vi "GetWirelessEndpointAuths.vi"(8 "error in (no error)":errorcluster) -> (0 "error out":errorcluster, 1 "found":bool, 3 "wireless endpoint auths":T1[](array[typedef]))   [LabVIEW 2017, in "GlobalConfiguration.lvlib"]
uses:
  <vilib>/addons/InsightCM/Utilities/GlobalConfiguration/GlobalConfiguration.lvlib
  <vilib>/addons/InsightCM/MessageBus/Base/controls/WirelessEndpointAuth.ctl
  <vilib>/addons/PointValueMap/subVIs/Point_Read_variant.vi
  <vilib>/addons/PointValueMap/subVIs/Point_Write_variant.vi
  <vilib>/addons/PointValueMap/PointValueMap.lvlib
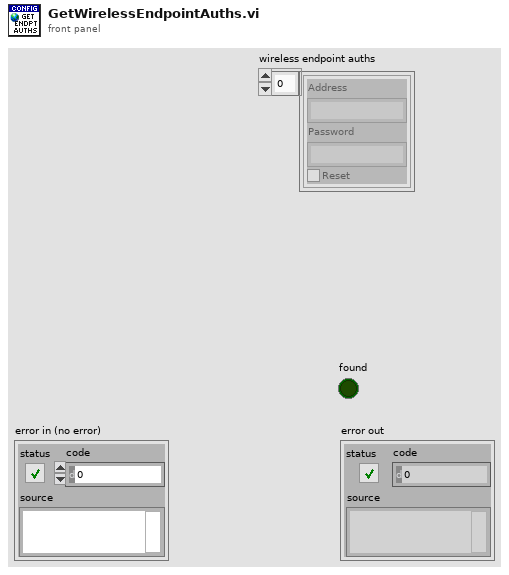
[diagram p1: front panel]
types:
  T1 = typedef "WirelessEndpointAuth.ctl" = cluster{"Address":string, "Password":string, "Reset":bool}
  T2 = typedef "PointValueMap.lvlib/PointMap.ctl" = refnum<data-value>
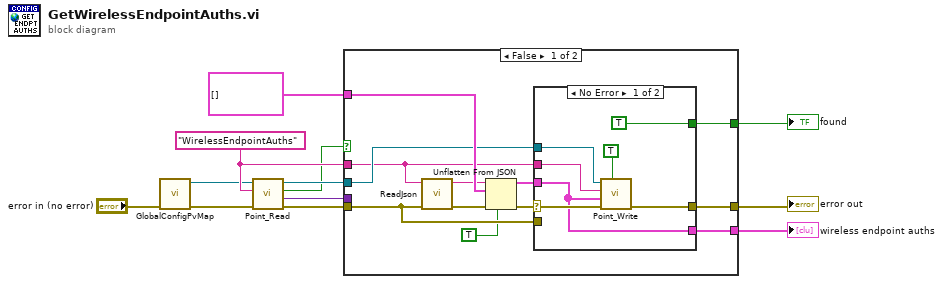
[diagram p0: block diagram]
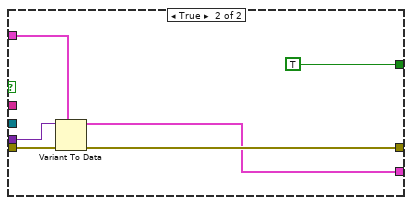
[diagram p3: hidden frame]
diagram:
  w10 = "WirelessEndpointAuths" ("Name")
  n1 = call <vilib>:"GlobalConfigPvMap.vi"("error in (no error)"="error in (no error)") -> ("error out"=w8:errorcluster, "global configuration map"=w9:T2)  [unwired: 9 in]
  n2 = call-poly <vilib>:"Point_Read.vi"("Error In"=w8, "Tag"=w10, "Map"=w9) -> ("Error Out"=w11:errorcluster, "Value"=w12:variant, "Found?"=w5:bool, "Map Out"=w7:T2)  [unwired: 3 in, 2 out]
  n3 = case shown="False" w5 {
    tunnel: [w15 w38] -> w3
    tunnel: [w16 w37] -> w1
    tunnel: [w20 TRUE] -> w4
    tunnel: w10 -> [w18 _]
    tunnel: T1[] [] -> [w23 w35]
    tunnel: w7 -> [w19 _]
    tunnel: w11 -> [w14 w34]
    tunnel: w12 -> [_ w33]
    frame False {
      n4 = call <vilib>:"ReadJson.vi"("error in (no error)"=w14, "json object"=w18) -> ("error out"=w24:errorcluster, "json string"=w22:string)  [unwired: 8 in]
      n5 = Unflatten From JSON(JSON string=w22, type and defaults=w23, default null elements? (F)=TRUE, error in (no error)=w24) -> (value=w17:T1[], error out=w21:errorcluster)  [unwired: 3 in]
      n6 = case shown="No Error" w21 {
        selector: w21 -> [w31 _]
        tunnel: [TRUE _] -> w20
        tunnel: w19 -> [w29 _]
        tunnel: w18 -> [w28 _]
        tunnel: w17 -> [w27 _]
        tunnel: [w27 _] -> w16
        tunnel: [w26 w32] -> w15
        tunnel: w14 -> [_ w32]
        frame No Error {
          n7 = call-poly <vilib>:"Point_Write.vi"("Auto Create?"=TRUE, "Error In"=w31, "Value"=w27, "Tag"=w28, "Map"=w29) -> ("Error Out"=w26:errorcluster)  [unwired: 5 in, 1 out]
        }
        frame Error {
        }
      }
    }
    frame True {
      n8 = Variant To Data(error in=w34, type=w35, Variant=w33) -> (data=w37:T1[], error out=w38:errorcluster)
    }
  }
  "error out" <- w3
  "found" <- w4
  "wireless endpoint auths" <- w1
